vi "MQTT_SubAck_Send.vi"(8 "error in (no error)":errorcluster, 9 "Granted QoS Levels":T1[](array[typedef]), 10 "Message ID":u16=10 format="%x", 11 "connection ID":refnum<k5>) -> (0 "error out":errorcluster, 2 "Suback Message":u8[](array[numeric]) format="%x", 3 "connection ID out":refnum<k5>)   [LabVIEW 2013, in "MQTT_Functions.lvlib"]
uses:
  MQTT_Functions.lvlib
  Controls/MessageType.ctl
  Controls/Retain_Flag.ctl
  Controls/DUP_Flag.ctl
  Controls/QoS.ctl
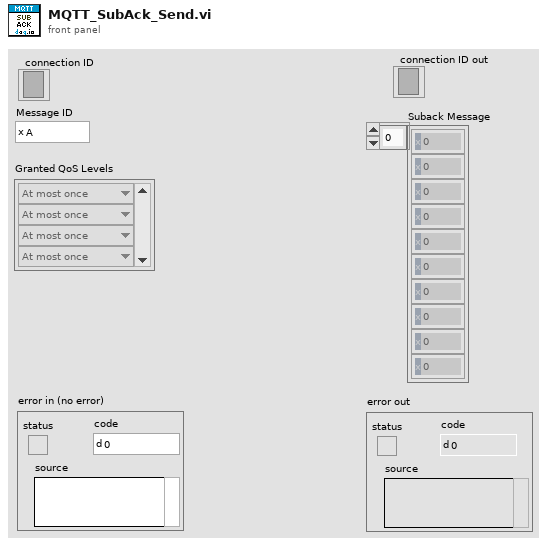
[diagram p1: front panel]
types:
  T1 = typedef "MQTT_Functions.lvlib/QoS.ctl" = enum8{"At most once", "At least once", "Exactly once", "Reserved"}
  T2 = typedef "MQTT_Functions.lvlib/DUP_Flag.ctl" = bool
  T3 = typedef "MQTT_Functions.lvlib/Retain_Flag.ctl" = bool
  T4 = typedef "MQTT_Functions.lvlib/MessageType.ctl" = enum32{"Reserved", "CONNECT", "CONNACK", "PUBLISH", "PUBACK", "PUBREC", "PUBREL", "PUBCOMP", "SUBSCRIBE", "SUBACK", "UNSUBSCRIBE", "UNSUBACK", "PINGREQ", "PINGRESP", "DISCONNECT", "Reserved2"}
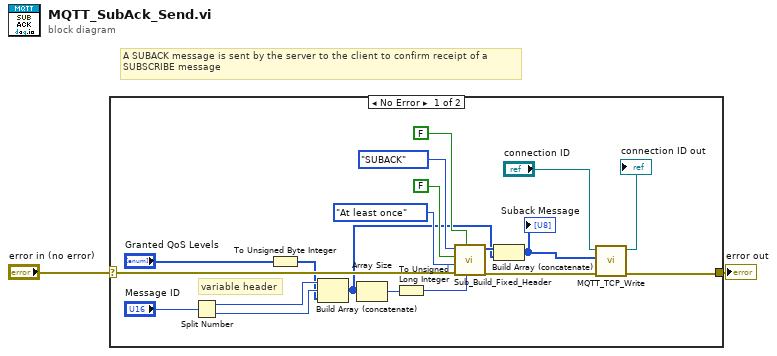
[diagram p0: block diagram]
diagram:
  # "A SUBACK message is sent by the server to the client to confirm receipt of a\nSUBSCRIBE message"
  n1 = case shown="No Error" "error in (no error)" {
    selector: "error in (no error)" -> [w13 w22]
    tunnel: [w5 w22] -> w1
    frame No Error {
      # "variable header"
      n2 = Split Number(x="Message ID") -> (hi(x)=w19:u8, lo(x)=w18:u8)
      n3 = To Unsigned Byte Integer(number="Granted QoS Levels") -> (unsigned 8bit integer=w8:u8[])
      n4 = Build Array (concatenate)(w19, w18, w8) -> (w12:u8[])
      n5 = Array Size(array=w12) -> (size(s)=w11:i32)
      n6 = To Unsigned Long Integer(number=w11) -> (unsigned 32bit integer=w10:u32)
      n7 = call "Sub_Build_Fixed_Header.vi"("Remaining Length"=w10, "Retain"=T3 FALSE, "error in (no error)"=w13, "QoS"=QoS."At least once", "DUP"=T2 FALSE, "MessageType"=MessageType."SUBACK") -> ("error out"=w4:errorcluster, "Fixed Header"=w20:u8[])  [unwired: 4 in]
      n8 = Build Array (concatenate)(w20, w12) -> (w3:u8[])
      "Suback Message" <- w3
      n9 = call "MQTT_TCP_Write.vi"("error in (no error)"=w4, "data in"=w3, "connection ID"="connection ID") -> ("error out"=w5:errorcluster, "connection ID out"=→"connection ID out":refnum<k5>)  [unwired: 6 in, 1 out]
    }
    frame Error {
    }
  }
  "error out" <- w1
